vi "6_Filtering.vi"(8 "error in (no error)":errorcluster) -> (0 "error out":errorcluster)   [LabVIEW 2014]
uses:
  SwabianInstruments.TimeTagger
panel:
  out "Test signal only on channel 2":dbl[](array[numeric])
  out "Test signal on channel 1 and 2":dbl[](array[numeric])
  # "counts / s"
  # "channel 1 (trigger)"
  # "counts / s"
  # "channel 2 (filtered)"
  # "channel 1 (trigger)"
  # "counts / s"
  # "channel 2 (filtered)"
  # "counts / s"
  # "Here, we have used the event filter between channel 1 and\nchannel 2 to suppress time tags on channel 2. The filter drops time tags on\nchannel 2 unless they were preceded by a tag on channel 1. First, since the tags are\nsimultaneous on both channels, but there is a finite jitter the count rate on channel 2\nis reduced by some amount. Now, as we disable the test signal on channel 1, all time\ntags on channel 2 are suppressed and a count rate of 0 is measured, even though the test\nsignal is active. The filtering is useful to tame signals with data rates > 8 MHz such as\nsynchronization signals from pulsed lasers in fluorescence lifetime measurements."
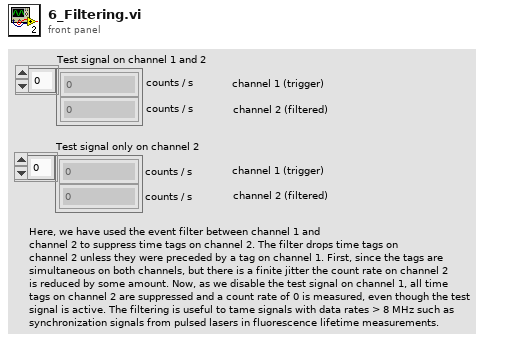
[diagram p1: front panel]
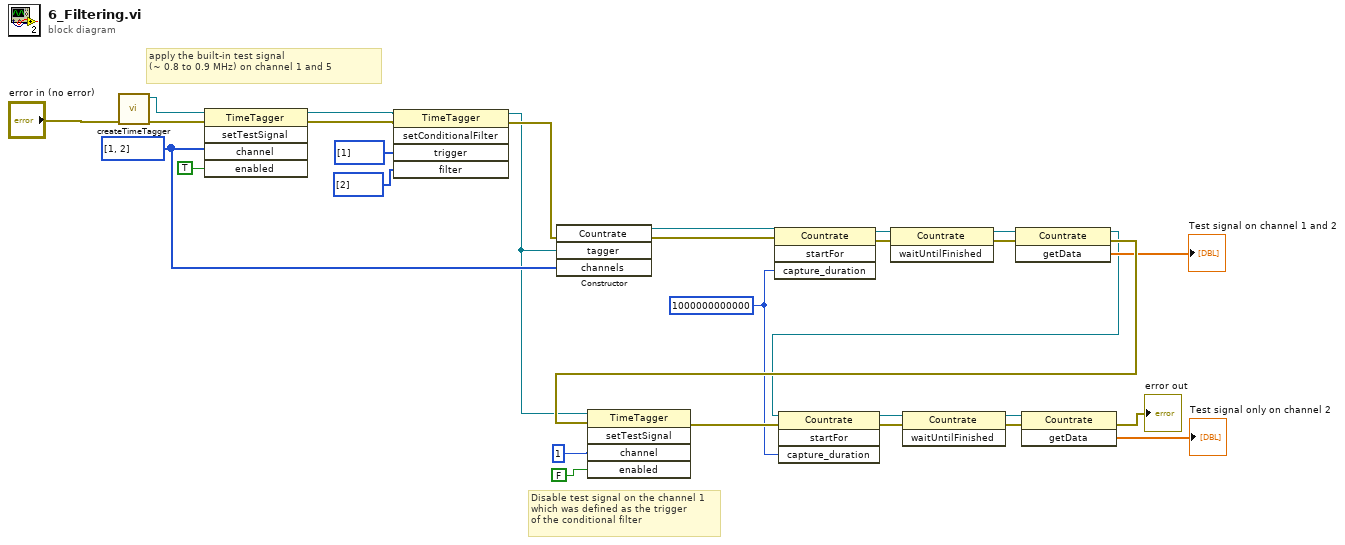
[diagram p0: block diagram]
diagram:
  w12 = i64 1000000000000 ("capture_duration")
  w17 = i32[] [1, 2]
  # "Disable test signal on the channel 1 \nwhich was defined as the trigger \nof the conditional filter"
  # "apply the built-in test signal\n(~ 0.8 to 0.9 MHz) on channel 1 and 5"
  n1 = call "createTimeTagger.vi"("error in (no error)"="error in (no error)") -> ("error out"=w20:errorcluster, "TimeTagger ref out"=w21:refnum<k24>)  [unwired: 9 in]
  n2 = invoke class="TimeTagger" method="setTestSignal"(reference=w21, error in=w20, "channel"=w17, "enabled"=TRUE) -> (reference out=w19:refnum<k24>, error out=w18:errorcluster)  [unwired: 1 in, 3 out]
  n3 = invoke class="TimeTagger" method="setConditionalFilter"(reference=w19, error in=w18, "trigger"=i32[] [1], "filter"=i32[] [2]) -> (reference out=w16:refnum<k24>, error out=w22:errorcluster)  [unwired: 1 in, 3 out]
  n4 = constructor class="Countrate"(error in=w22, "tagger"=w16, "channels"=w17) -> (reference out=w14:refnum<k24>, error out=w15:errorcluster)  [unwired: 2 in, 3 out]
  n5 = invoke class="Countrate" method="startFor"(reference=w14, error in=w15, "capture_duration"=w12) -> (reference out=w9:refnum<k24>, error out=w10:errorcluster)  [unwired: 1 in, 2 out]
  n6 = invoke class="Countrate" method="waitUntilFinished"(reference=w9, error in=w10) -> (reference out=w8:refnum<k24>, error out=w7:errorcluster)  [unwired: 1 in, 1 out]
  n7 = invoke class="Countrate" method="getData"(reference=w8, error in=w7) -> (reference out=w11:refnum<k24>, error out=w27:errorcluster, "getData"=→"Test signal on channel 1 and 2":dbl[])  [unwired: 1 in]
  n8 = invoke class="TimeTagger" method="setTestSignal"(reference=w16, error in=w27, "channel"=1, "enabled"=FALSE) -> (error out=w13:errorcluster)  [unwired: 1 in, 4 out]
  n9 = invoke class="Countrate" method="startFor"(reference=w11, error in=w13, "capture_duration"=w12) -> (reference out=w4:refnum<k24>, error out=w3:errorcluster)  [unwired: 1 in, 2 out]
  n10 = invoke class="Countrate" method="waitUntilFinished"(reference=w4, error in=w3) -> (reference out=w6:refnum<k24>, error out=w5:errorcluster)  [unwired: 1 in, 1 out]
  n11 = invoke class="Countrate" method="getData"(reference=w6, error in=w5) -> (error out=→"error out":errorcluster, "getData"=→"Test signal only on channel 2":dbl[])  [unwired: 1 in, 1 out]
